vi "File - Valid Key Name.vi"(4 "Key Name In":string) -> (1 "Key Name Out":string)   [LabVIEW 2020]
doc: "Ensures an INI key name contains valid characters only, removes spaces."
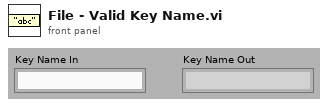
[diagram p1: front panel]
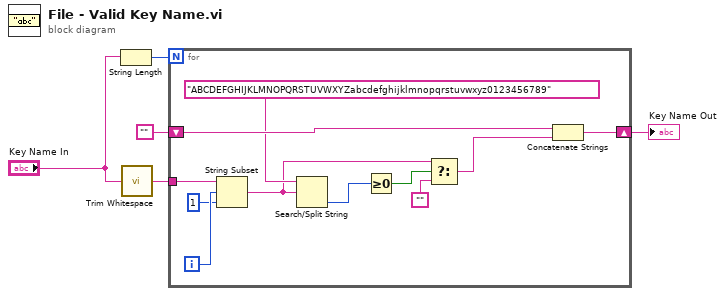
[diagram p0: block diagram]
diagram:
  n1 = String Length(string="Key Name In") -> (length=w2:i32)
  n2 = call <vilib>:"Trim Whitespace.vi"("string"="Key Name In") -> ("trimmed string"=w3:string)  [unwired: 1 in]
  n3 = for {
    N: w2 -> [_]
    tunnel: w3 -> [w16]
    shift-right: [w12] -> w4
    shift-left: "" -> [w13]
    i -> [w15]
    n4 = String Subset(string=w16, offset (0)=w15, length (rest)=1 ("length (rest)")) -> (substring=w8:string)
    n5 = Search/Split String(string="ABCDEFGHIJKLMNOPQRSTUVWXYZabcdefghijklmnopqrstuvwxyz0123456789", search string/char (-)=w8) -> (offset of match=w10:i32)  [unwired: 1 in, 2 out]
    n6 = Greater Or Equal To 0?(x=w10) -> (x >= 0?=w7:bool)
    n7 = Select(t=w8, s=w7, f="") -> (s? t:f=w9:string)
    n8 = Concatenate Strings(w13, w9) -> (w12:string)
  }
  "Key Name Out" <- w4
